vi "TreeItem.Property.Set.vi"(4 "Set String as Binary":bool, 6 "Custom Device Path":string, 8 "error in (no error)":errorcluster, 9 "Value":variant, 10 "Property Name":string, 11 "BaseNodeType":refnum<k24>) -> (0 "error out":errorcluster, 1 "Replaced":bool, 3 "BaseNodeType":refnum<k24>)   [LabVIEW 2016, in "Advanced System Definition.lvlib"]
doc: "Saves the new values/items into their corresponding position within the Custom Device Hierarchy according to their corresponding data type."
uses:
  SysDef API/Advanced System Definition.lvlib
  NationalInstruments.VeriStand.SystemStorage
  _Types/Property.DependentFile.ctl
  NationalInstruments.VeriStand
  <vilib>/NI Veristand/Custom Device API/Custom Device Item Ref.ctl
  NationalInstruments.VeriStand.SystemDefinitionAPI
  <vilib>/Utility/VariantDataType/VariantType.lvlib
  <vilib>/NI VeriStand/Custom Device API/Custom Device API.lvlib
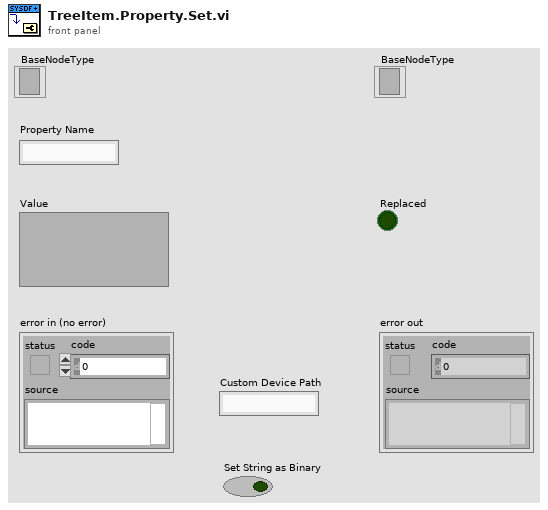
[diagram p1: front panel]
types:
  T1 = typedef "Advanced System Definition.lvlib/Property.DependentFile.ctl" = cluster{"Original Path":path, "Version":string, "RTDestination":path, "ForceDownload":bool, "SupportedTarget":string, "MD5":string}
  T2 = typedef "Custom Device API.lvlib/Custom Device Item Ref.ctl" = u64
  T3 = typedef "VariantType.lvlib/Type.ctl" = enum8{"Invalid Type", "Void", "I8", "I16", "I32", "I64", "U8", "U16", "U32", "U64", "Single Float", "Double Float", "Extended Float", "Single Complex", "Double Complex", "Extended Complex", "Enum U8", "Enum U16", "Enum U32", "Enum U64", "Single Float With Unit", "Double Float With Unit", "Extended Float With Unit", "Single Complex with Unit", "Double Complex with Unit", "Extended Complex with Unit", "Boolean", "String", "Path", "Picture", "Tag", "Array", "Cluster", "Variant", "LV Variant", "Waveform", "Timestamp", "Digital Waveform", "Digital Data", "ExpressData", "Refnum", "External Data", "VI", "Poly VI", "LabVIEW Class Instance", "Fixed Point"}
  T4 = typedef "Advanced System Definition.lvlib/Property.Dictionary.ctl" = cluster{"Dictionary Type":string, "Keys":string[], "Values":variant[]}
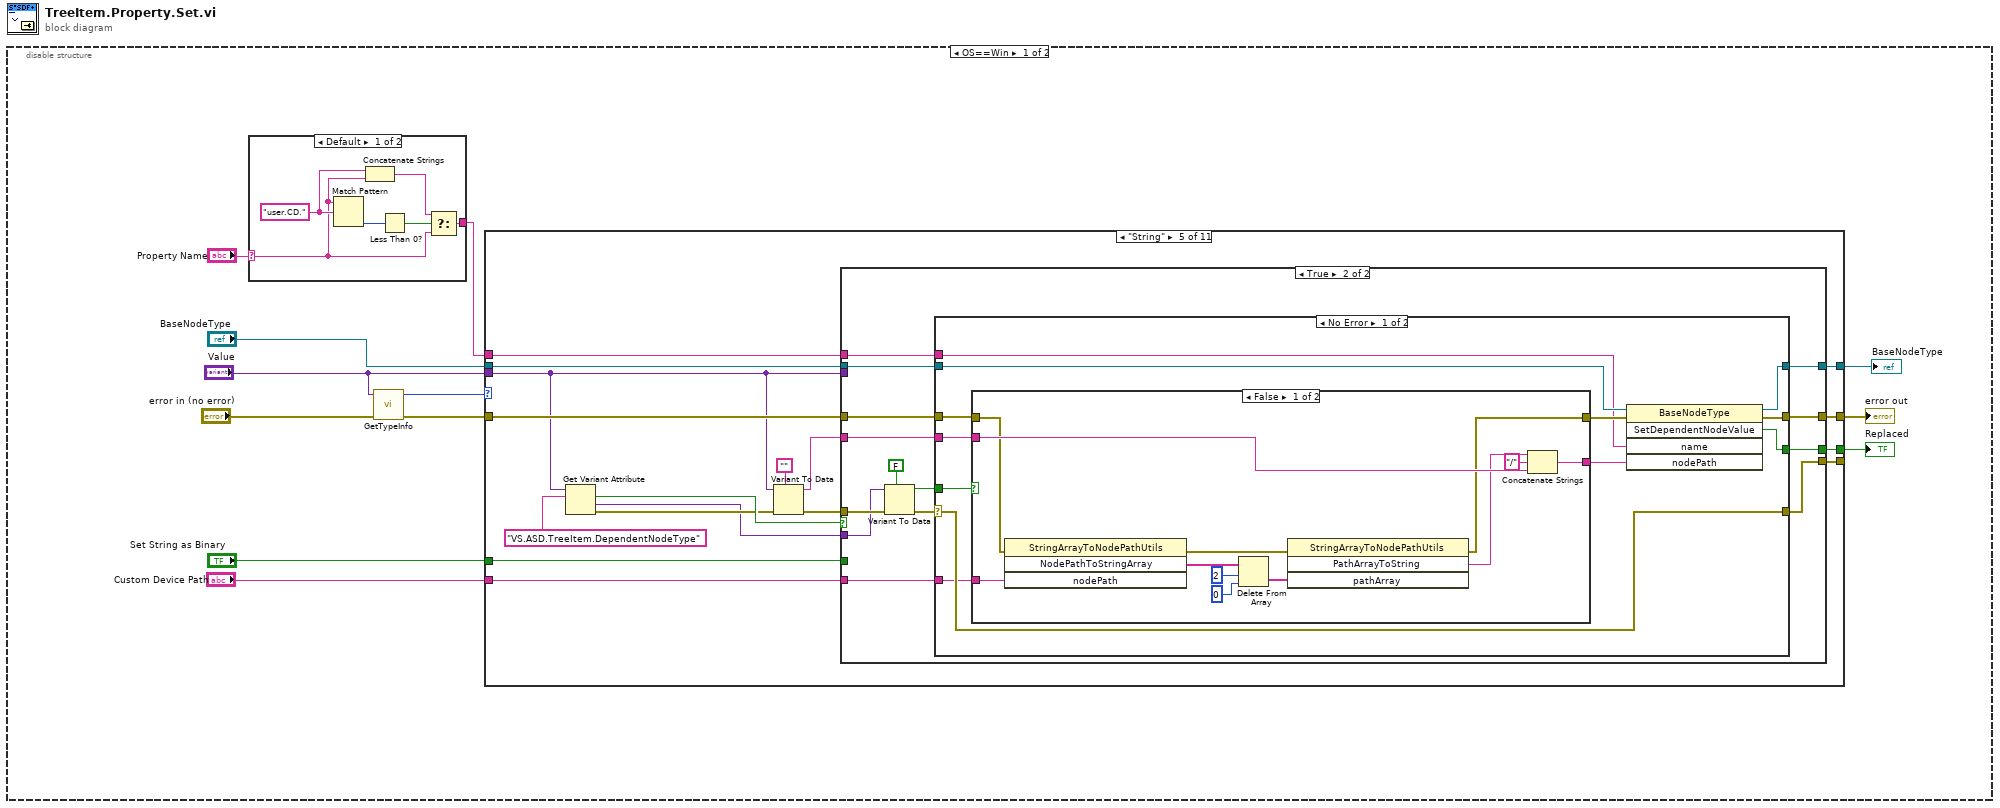
[diagram p0: block diagram]
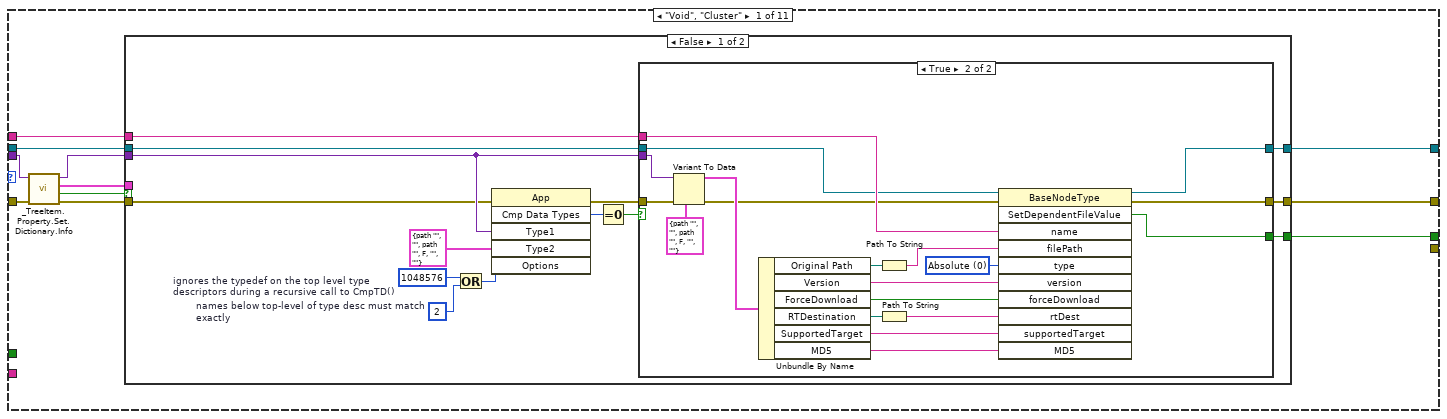
[diagram p3: hidden frame]
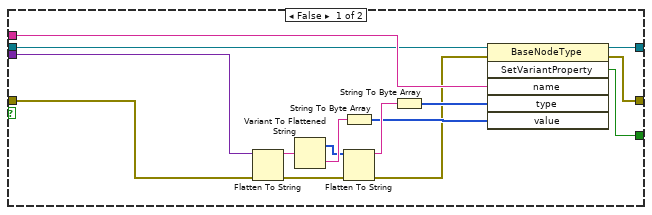
[diagram p4: hidden frame]
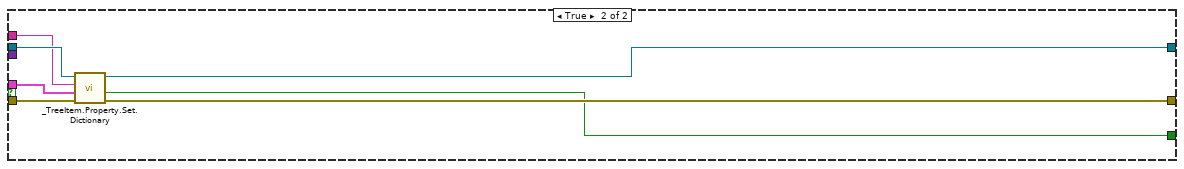
[diagram p5: hidden frame]
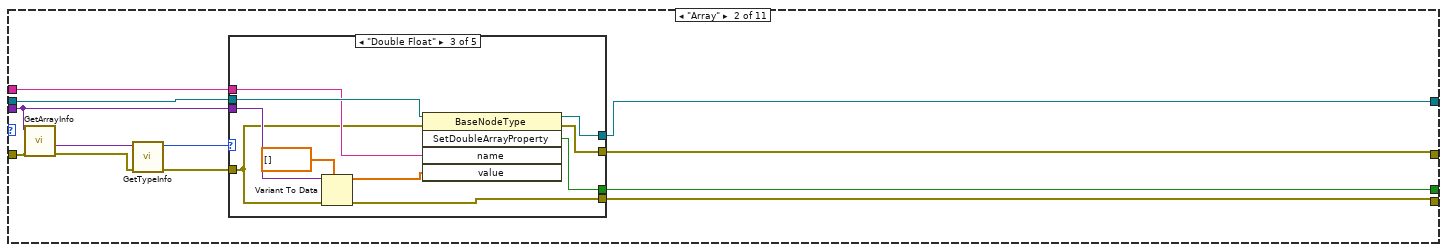
[diagram p6: hidden frame]
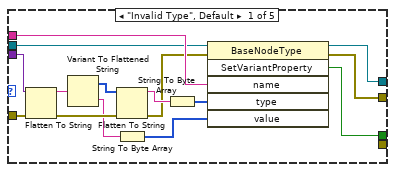
[diagram p7: hidden frame]
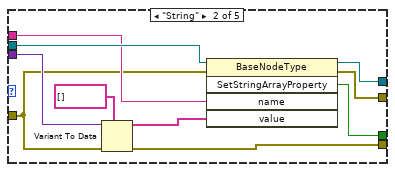
[diagram p8: hidden frame]
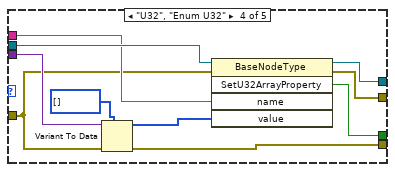
[diagram p9: hidden frame]
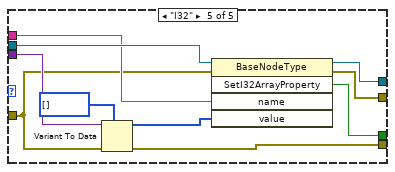
[diagram p10: hidden frame]
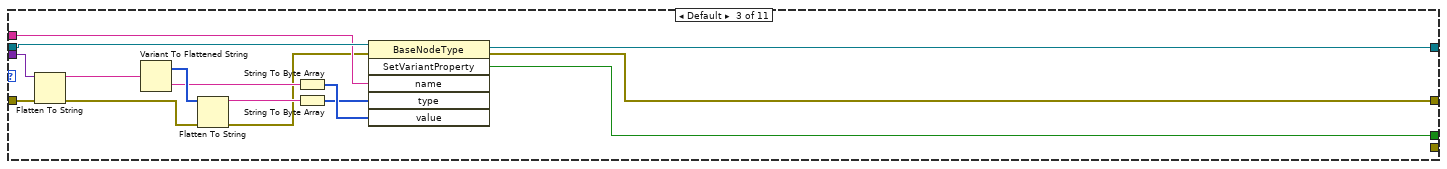
[diagram p11: hidden frame]
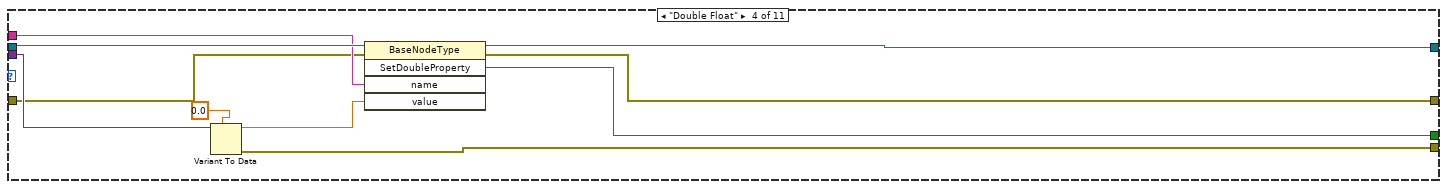
[diagram p12: hidden frame]
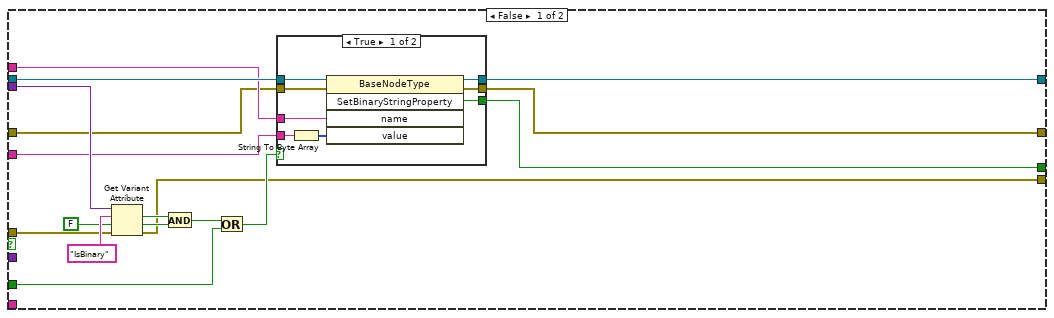
[diagram p13: hidden frame]
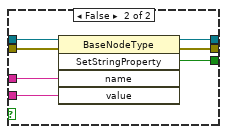
[diagram p14: hidden frame]
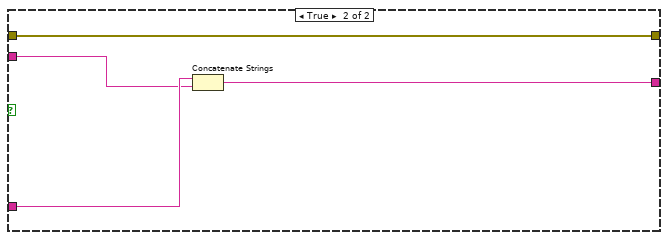
[diagram p15: hidden frame]
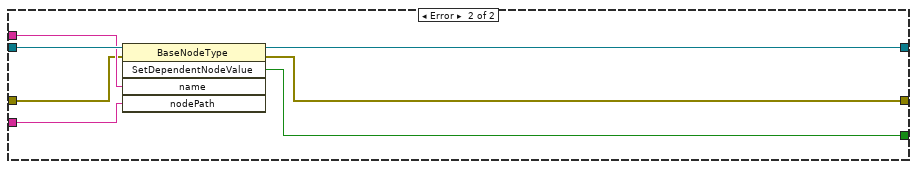
[diagram p16: hidden frame]
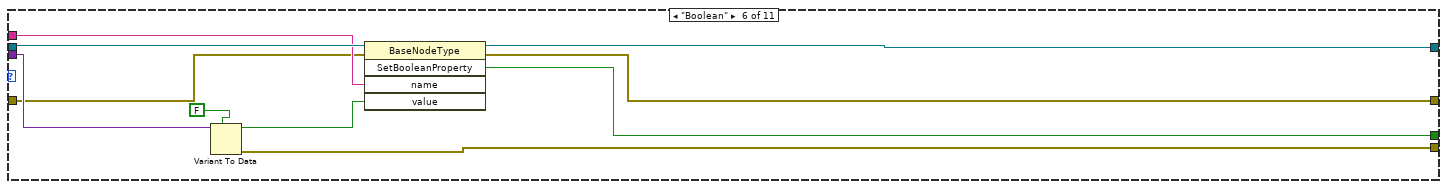
[diagram p17: hidden frame]
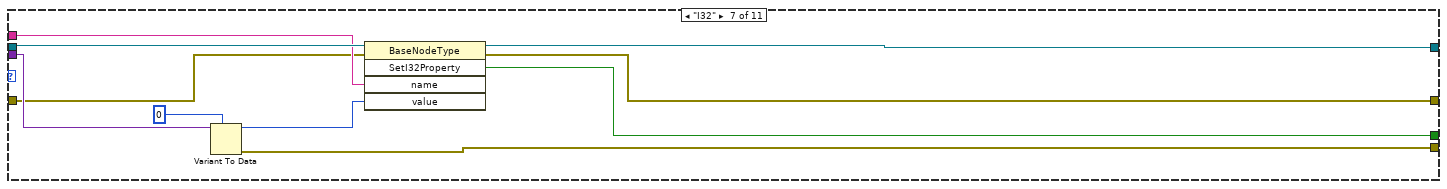
[diagram p18: hidden frame]
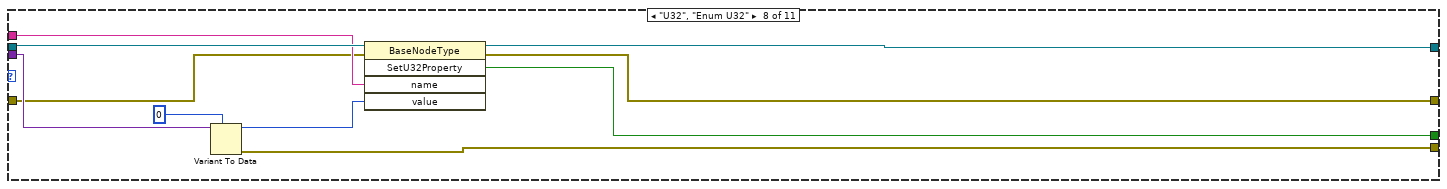
[diagram p19: hidden frame]
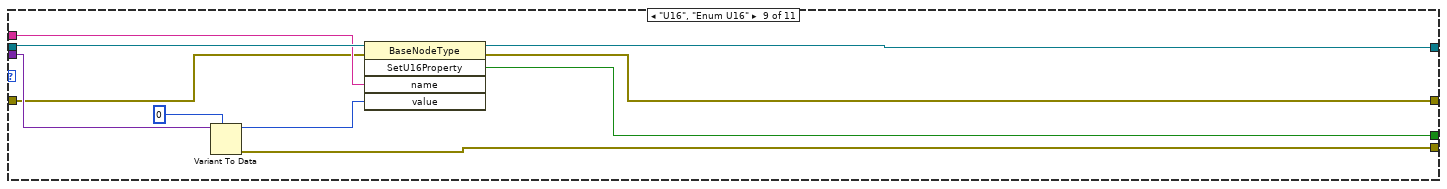
[diagram p20: hidden frame]
diagram:
  n1 = disable-structure shown="OS==Win" {
    frame condition #0 (active) {
      n2 = case shown="Default" "Property Name" {
        selector: "Property Name" -> [w13 w19]
        tunnel: [w14 w19] -> w3
        frame Default {
          w15 = "user.CD." ("regular expression")
          n3 = Match Pattern(string=w13, regular expression=w15) -> (offset past match=w18:i32)  [unwired: 1 in, 3 out]
          n4 = Concatenate Strings(w15, w13) -> (w16:string)
          n5 = Less Than 0?(x=w18) -> (x < 0?=w17:bool)
          n6 = Select(t=w16, s=w17, f=w13) -> (s? t:f=w14:string)
        }
        frame "Value Table" {
        }
      }
      n7 = call <vilib>:"GetTypeInfo.vi"("error in (no error)"="error in (no error)", "Variant"="Value") -> ("error out"=w8:errorcluster, "Type Enum"=w12:T3)  [unwired: 5 in, 3 out]
      n8 = case shown="\"String\"" w12 {
        tunnel: "BaseNodeType" -> [w29 w92 w167 w174 w193 w282 w292 w302 w312 w319 w356]
        tunnel: w8 -> [w24 w97 w157 w172 w186 w280 w290 w300 w310 w322 w355]
        tunnel: [w28 w90 w165 w171 w191 w279 w289 w299 w309 w318 w351] -> w11
        tunnel: w3 -> [w30 w91 w166 w173 w192 w281 w291 w301 w311 w320 w353]
        tunnel: "Value" -> [w25 w86 w156 w177 w181 w285 w295 w305 w315 w328 w359]
        tunnel: [w27 w89 w164 w170 w190 w278 w288 w298 w308 w316 w350] -> w10
        tunnel: [_ w88 _ w175 w194 w283 w293 w303 w313 _ w354] -> _
        tunnel: [w26 w87 w163 w168 w189 w276 w286 w296 w306 w317 w349] -> w5
        tunnel: "Set String as Binary" -> [_ _ _ _ w188 _ _ _ _ _ _]
        tunnel: "Custom Device Path" -> [_ _ _ _ w178 _ _ _ _ _ _]
        frame "Void", "Cluster" {
          n9 = call "_TreeItem.Property.Set.Dictionary.Info.vi"("error in"=w24, "Variant"=w25) -> ("error out"=w23:errorcluster, "Dictionary?"=w22:bool, "Dictionary Info"=w21:T4, "Variant out"=w20:variant)  [unwired: 6 in]
          n10 = case shown="False" w22 {
            tunnel: w30 -> [w44 w84]
            tunnel: w29 -> [w43 w85]
            tunnel: [w42 w82] -> w28
            tunnel: [w41 w80] -> w27
            tunnel: [w40 w81] -> w26
            tunnel: w20 -> [w35 _]
            tunnel: w23 -> [w32 w83]
            tunnel: w21 -> [_ w79]
            frame False {
              w38 = 2  # names below top-level of type desc must match exactly
              w37 = 1048576  # ignores the typedef on the top level type descriptors during a recursive call to CmpTD()
              n11 = Or(x=w37, y=w38) -> (x .or. y?=w39:i32)
              n12 = invoke class="App" method="Cmp Data Types"(error in=w32, "Type1"=w35, "Type2"=T1 {"Original Path"=path "", "Version"="", "RTDestination"=path "", "ForceDownload"=FALSE, "SupportedTarget"="", "MD5"=""} ("OptionalInfo"), "Options"=w39) -> (error out=w31:errorcluster, "Compare Data Types"=w36:i32)  [unwired: 2 in, 4 out]
              n13 = Equal To 0?(x=w36) -> (x = 0?=w33:bool)
              n14 = case shown="True" w33 {
                tunnel: w44 -> [w59 w73]
                tunnel: w43 -> [w58 w71]
                tunnel: [w57 w62] -> w42
                tunnel: [w56 w61] -> w41
                tunnel: [w55 w70] -> w40
                tunnel: w31 -> [w49 w77]
                tunnel: w35 -> [w45 w78]
                frame False {
                  n15 = Flatten To String(anything=w45, error in (no error)=w49) -> (data string=w51:string, error out=w50:errorcluster)  [unwired: 2 in, 1 out]
                  n16 = Variant To Flattened String(Variant=w51) -> (data string=w54:string, 1:w52:i16[])
                  n17 = String To Byte Array(string=w54) -> (unsigned byte array=w48:u8[])
                  n18 = Flatten To String(anything=w52, error in (no error)=w50) -> (data string=w53:string, error out=w46:errorcluster)  [unwired: 2 in, 1 out]
                  n19 = String To Byte Array(string=w53) -> (unsigned byte array=w47:u8[])
                  n20 = invoke class="BaseNodeType" method="SetVariantProperty"(reference=w58, error in=w46, "name"=w59, "type"=w47, "value"=w48) -> (reference out=w55:refnum<k24>, error out=w57:errorcluster, "SetVariantProperty"=w56:bool)  [unwired: 1 in, 3 out]
                }
                frame True {
                  w60 = 0 items=["Absolute", "Relative", "ToCommonDocDir", "ToApplicationDataDir"] ("type")
                  n21 = Variant To Data(error in=w77, type=T1 {"Original Path"=path "", "Version"="", "RTDestination"=path "", "ForceDownload"=FALSE, "SupportedTarget"="", "MD5"=""} ("OptionalInfo"), Variant=w78) -> (data=w74:T1, error out=w63:errorcluster)
                  n22 = Unbundle By Name(w74) -> ("Original Path"=w72:path, "Version"=w68:string, "ForceDownload"=w67:bool, "RTDestination"=w75:path, "SupportedTarget"=w65:string, "MD5"=w64:string)
                  n23 = Path To String(path=w72) -> (string=w69:string)
                  n24 = Path To String(path=w75) -> (string=w66:string)
                  n25 = invoke class="BaseNodeType" method="SetDependentFileValue"(reference=w71, error in=w63, "name"=w73, "filePath"=w69, "type"=w60, "version"=w68, "forceDownload"=w67, "rtDest"=w66, "supportedTarget"=w65, "MD5"=w64) -> (reference out=w70:refnum<k24>, error out=w62:errorcluster, "SetDependentFileValue"=w61:bool)  [unwired: 1 in, 8 out]
                }
              }
            }
            frame True {
              n26 = call "_TreeItem.Property.Set.Dictionary.vi"("error in (no error)"=w83, "Dictionary"=w79, "Property Name"=w84, "BaseNodeType"=w85) -> ("error out"=w82:errorcluster, "Replaced"=w80:bool, "BaseNodeType out"=w81:refnum<k24>)  [unwired: 5 in]
            }
          }
        }
        frame "Array" {
          n27 = call <vilib>:"GetArrayInfo.vi"("error in (no error)"=w97, "Variant"=w86) -> ("error out"=w95:errorcluster, "ArrayElement"=w96:variant)  [unwired: 6 in, 2 out]
          n28 = call <vilib>:"GetTypeInfo.vi"("error in (no error)"=w95, "Variant"=w96) -> ("error out"=w93:errorcluster, "Type Enum"=w94:T3)  [unwired: 5 in, 3 out]
          n29 = case shown="\"Double Float\"" w94 {
            tunnel: w93 -> [w99 w115 w127 w136 w147]
            tunnel: w86 -> [w100 w122 w132 w142 w152]
            tunnel: w92 -> [w111 w119 w130 w140 w150]
            tunnel: w91 -> [w112 w117 w128 w138 w148]
            tunnel: [w110 w118 w129 w139 w149] -> w87
            tunnel: [w109 w113 w125 w134 w145] -> w90
            tunnel: [w108 w114 w126 w135 w146] -> w89
            tunnel: [_ w120 w131 w141 w151] -> w88
            frame "Invalid Type", Default {
              n30 = Flatten To String(anything=w100, error in (no error)=w99) -> (data string=w106:string, error out=w107:errorcluster)  [unwired: 2 in, 1 out]
              n31 = Variant To Flattened String(Variant=w106) -> (data string=w103:string, 1:w105:i16[])
              n32 = Flatten To String(anything=w105, error in (no error)=w107) -> (data string=w104:string, error out=w98:errorcluster)  [unwired: 2 in, 1 out]
              n33 = String To Byte Array(string=w103) -> (unsigned byte array=w101:u8[])
              n34 = String To Byte Array(string=w104) -> (unsigned byte array=w102:u8[])
              n35 = invoke class="BaseNodeType" method="SetVariantProperty"(reference=w111, error in=w98, "name"=w112, "type"=w102, "value"=w101) -> (reference out=w110:refnum<k24>, error out=w109:errorcluster, "SetVariantProperty"=w108:bool)  [unwired: 1 in, 3 out]
            }
            frame "String" {
              n36 = Variant To Data(error in=w115, type=string[] [], Variant=w122) -> (data=w116:string[], error out=w120:errorcluster)
              n37 = invoke class="BaseNodeType" method="SetStringArrayProperty"(reference=w119, error in=w115, "name"=w117, "value"=w116) -> (reference out=w118:refnum<k24>, error out=w113:errorcluster, "SetStringArrayProperty"=w114:bool)  [unwired: 1 in, 2 out]
            }
            frame "Double Float" {
              n38 = Variant To Data(error in=w127, type=dbl[] [], Variant=w132) -> (data=w123:dbl[], error out=w131:errorcluster)
              n39 = invoke class="BaseNodeType" method="SetDoubleArrayProperty"(reference=w130, error in=w127, "name"=w128, "value"=w123) -> (reference out=w129:refnum<k24>, error out=w125:errorcluster, "SetDoubleArrayProperty"=w126:bool)  [unwired: 1 in, 2 out]
            }
            frame "U32", "Enum U32" {
              n40 = Variant To Data(error in=w136, type=u32[] [], Variant=w142) -> (data=w137:u32[], error out=w141:errorcluster)
              n41 = invoke class="BaseNodeType" method="SetU32ArrayProperty"(reference=w140, error in=w136, "name"=w138, "value"=w137) -> (reference out=w139:refnum<k24>, error out=w134:errorcluster, "SetU32ArrayProperty"=w135:bool)  [unwired: 1 in, 2 out]
            }
            frame "I32" {
              n42 = Variant To Data(error in=w147, type=i32[] [], Variant=w152) -> (data=w143:i32[], error out=w151:errorcluster)
              n43 = invoke class="BaseNodeType" method="SetI32ArrayProperty"(reference=w150, error in=w147, "name"=w148, "value"=w143) -> (reference out=w149:refnum<k24>, error out=w145:errorcluster, "SetI32ArrayProperty"=w146:bool)  [unwired: 1 in, 2 out]
            }
          }
        }
        frame Default {
          n44 = Flatten To String(anything=w156, error in (no error)=w157) -> (data string=w161:string, error out=w162:errorcluster)  [unwired: 2 in, 1 out]
          n45 = Variant To Flattened String(Variant=w161) -> (data string=w158:string, 1:w160:i16[])
          n46 = Flatten To String(anything=w160, error in (no error)=w162) -> (data string=w159:string, error out=w155:errorcluster)  [unwired: 2 in, 1 out]
          n47 = String To Byte Array(string=w158) -> (unsigned byte array=w154:u8[])
          n48 = String To Byte Array(string=w159) -> (unsigned byte array=w153:u8[])
          n49 = invoke class="BaseNodeType" method="SetVariantProperty"(reference=w167, error in=w155, "name"=w166, "type"=w153, "value"=w154) -> (reference out=w163:refnum<k24>, error out=w165:errorcluster, "SetVariantProperty"=w164:bool)  [unwired: 1 in, 3 out]
        }
        frame "Double Float" {
          n50 = Variant To Data(type=0.0, Variant=w177) -> (data=w169:dbl, error out=w175:errorcluster)  [unwired: 1 in]
          n51 = invoke class="BaseNodeType" method="SetDoubleProperty"(reference=w174, error in=w172, "name"=w173, "value"=w169) -> (reference out=w168:refnum<k24>, error out=w171:errorcluster, "SetDoubleProperty"=w170:bool)  [unwired: 1 in, 2 out]
        }
        frame "String" {
          n52 = Get Variant Attribute(Variant=w181, name="VS.ASD.TreeItem.DependentNodeType") -> (found=w185:bool, value=w179:variant, error out=w183:errorcluster)  [unwired: 2 in, 1 out]
          n53 = Variant To Data(error in=w183, type="", Variant=w181) -> (data=w180:string, error out=w182:errorcluster)
          n54 = case shown="True" w185 {
            tunnel: [w195 w229] -> w194
            tunnel: w193 -> [w211 w240]
            tunnel: w192 -> [w210 w238]
            tunnel: [w209 w236] -> w191
            tunnel: [w208 w235] -> w190
            tunnel: [w207 w239] -> w189
            tunnel: w188 -> [w201 _]
            tunnel: w181 -> [w199 _]
            tunnel: w182 -> [w198 w233]
            tunnel: w186 -> [w197 w237]
            tunnel: w180 -> [w196 w234]
            tunnel: w179 -> [_ w232]
            tunnel: w178 -> [_ w227]
            frame False {
              n55 = Get Variant Attribute(Variant=w199, name="IsBinary", default value (empty Variant)=FALSE ("Set String as Binary"), error in=w198) -> (found=w204:bool, value=w205:bool, error out=w195:errorcluster)  [unwired: 1 out]
              n56 = And(x=w204, y=w205) -> (x .and. y?=w206:bool)
              n57 = Or(x=w206, y=w201) -> (x .or. y?=w200:bool)
              n58 = case shown="True" w200 {
                tunnel: w211 -> [w219 w226]
                tunnel: w210 -> [w218 w225]
                tunnel: w197 -> [w217 w224]
                tunnel: [w216 w223] -> w209
                tunnel: [w215 w222] -> w208
                tunnel: w196 -> [w214 w221]
                tunnel: [w213 w220] -> w207
                frame True {
                  n59 = String To Byte Array(string=w214) -> (unsigned byte array=w212:u8[])
                  n60 = invoke class="BaseNodeType" method="SetBinaryStringProperty"(reference=w219, error in=w217, "name"=w218, "value"=w212) -> (reference out=w213:refnum<k24>, error out=w216:errorcluster, "SetBinaryStringProperty"=w215:bool)  [unwired: 1 in, 2 out]
                }
                frame False {
                  n61 = invoke class="BaseNodeType" method="SetStringProperty"(reference=w226, error in=w224, "name"=w225, "value"=w221) -> (reference out=w220:refnum<k24>, error out=w223:errorcluster, "SetStringProperty"=w222:bool)  [unwired: 1 in, 2 out]
                }
              }
            }
            frame True {
              n62 = Variant To Data(error in=w233, type=FALSE, Variant=w232) -> (data=w228:bool, error out=w231:errorcluster)
              n63 = case shown="No Error" w231 {
                selector: w231 -> [w252 _]
                tunnel: w240 -> [w245 w275]
                tunnel: [w246 w274] -> w239
                tunnel: w238 -> [w244 w273]
                tunnel: w237 -> [w251 w272]
                tunnel: [w247 w271] -> w236
                tunnel: [w242 w270] -> w235
                tunnel: w234 -> [w250 w269]
                tunnel: [w252 _] -> w229
                tunnel: w228 -> [w249 _]
                tunnel: w227 -> [w241 _]
                frame No Error {
                  n64 = case shown="False" w249 {
                    tunnel: w241 -> [w260 w268]
                    tunnel: w250 -> [w259 w267]
                    tunnel: [w257 w266] -> w243
                    tunnel: w251 -> [w253 w265]
                    tunnel: [w254 w265] -> w248
                    frame False {
                      n65 = invoke class="StringArrayToNodePathUtils" method="NodePathToStringArray"(error in=w253, "nodePath"=w260) -> (error out=w261:errorcluster, "NodePathToStringArray"=w264:string[])  [unwired: 2 in, 2 out]
                      n66 = Delete From Array(array=w264, length=2, index=0) -> (deleted portion=w255:string[])  [unwired: 1 out]
                      n67 = invoke class="StringArrayToNodePathUtils" method="PathArrayToString"(error in=w261, "pathArray"=w255) -> (error out=w254:errorcluster, "PathArrayToString"=w258:string)  [unwired: 2 in, 2 out]
                      n68 = Concatenate Strings(w258, "/" ("string"), w259) -> (w257:string)
                    }
                    frame True {
                      n69 = Concatenate Strings(w268, w267) -> (w266:string)
                    }
                  }
                  n70 = invoke class="BaseNodeType" method="SetDependentNodeValue"(reference=w245, error in=w248, "name"=w244, "nodePath"=w243) -> (reference out=w246:refnum<k24>, error out=w247:errorcluster, "SetDependentNodeValue"=w242:bool)  [unwired: 1 in, 2 out]
                }
                frame Error {
                  n71 = invoke class="BaseNodeType" method="SetDependentNodeValue"(reference=w275, error in=w272, "name"=w273, "nodePath"=w269) -> (reference out=w274:refnum<k24>, error out=w271:errorcluster, "SetDependentNodeValue"=w270:bool)  [unwired: 1 in, 2 out]
                }
              }
            }
          }
        }
        frame "Boolean" {
          n72 = Variant To Data(type=FALSE, Variant=w285) -> (data=w277:bool, error out=w283:errorcluster)  [unwired: 1 in]
          n73 = invoke class="BaseNodeType" method="SetBooleanProperty"(reference=w282, error in=w280, "name"=w281, "value"=w277) -> (reference out=w276:refnum<k24>, error out=w279:errorcluster, "SetBooleanProperty"=w278:bool)  [unwired: 1 in, 2 out]
        }
        frame "I32" {
          n74 = Variant To Data(type=0, Variant=w295) -> (data=w287:i32, error out=w293:errorcluster)  [unwired: 1 in]
          n75 = invoke class="BaseNodeType" method="SetI32Property"(reference=w292, error in=w290, "name"=w291, "value"=w287) -> (reference out=w286:refnum<k24>, error out=w289:errorcluster, "SetI32Property"=w288:bool)  [unwired: 1 in, 2 out]
        }
        frame "U32", "Enum U32" {
          n76 = Variant To Data(type=u32 0, Variant=w305) -> (data=w297:u32, error out=w303:errorcluster)  [unwired: 1 in]
          n77 = invoke class="BaseNodeType" method="SetU32Property"(reference=w302, error in=w300, "name"=w301, "value"=w297) -> (reference out=w296:refnum<k24>, error out=w299:errorcluster, "SetU32Property"=w298:bool)  [unwired: 1 in, 2 out]
        }
        frame "U16", "Enum U16" {
          n78 = Variant To Data(type=u16 0, Variant=w315) -> (data=w307:u16, error out=w313:errorcluster)  [unwired: 1 in]
          n79 = invoke class="BaseNodeType" method="SetU16Property"(reference=w312, error in=w310, "name"=w311, "value"=w307) -> (reference out=w306:refnum<k24>, error out=w309:errorcluster, "SetU16Property"=w308:bool)  [unwired: 1 in, 2 out]
        }
        frame "U64" {
          # "This is the legacy dependent node format;\ndependent node properties are now serialized\nas strings containing the node path with a variant\nattribute to indicate they are dependent nodes."
          n80 = Variant To Data(error in=w322, type=u64 0, Variant=w328) -> (data=w323:u64)  [unwired: 1 out]
          n81 = Equal?(x=T2 18446744073709551615 ("Dependent Node Ref"), y=w323) -> (x = y?=w325:bool)
          n82 = case shown="False" w325 {
            tunnel: [w338 ""] -> w324
            tunnel: w323 -> [w331 _]
            tunnel: w322 -> [w330 w347]
            tunnel: [w329 w347] -> w321
            frame False {
              n83 = constructor class="NodeIDUtil"(error in=w330) -> (reference out=w334:refnum<k24>, error out=w335:errorcluster)  [unwired: 2 in, 1 out]
              n84 = invoke class="NodeIDUtil" method="IDToBaseNode"(reference=w334, error in=w335, "nodeID"=w331) -> (reference out=w337:refnum<k24>, error out=w336:errorcluster, "IDToBaseNode"=w332:refnum<k24>)  [unwired: 1 in, 1 out]
              n85 = Close Reference(reference=w337, error in (no error)=w336) -> (error out=w333:errorcluster)
              n86 = case shown="No Error" w333 {
                selector: w333 -> [w340 w345]
                tunnel: w332 -> [w344 _]
                tunnel: [w343 ""] -> w338
                tunnel: [w339 w345] -> w329
                frame No Error {
                  n87 = property class="BaseNode"(reference=w344, error in=w340) -> (reference out=w341:refnum<k24>, error out=w342:errorcluster, "NodePath"=w343:string)
                  n88 = Close Reference(reference=w341, error in (no error)=w342) -> (error out=w339:errorcluster)
                }
                frame Error {
                }
              }
            }
            frame True {
              # "If user call this with an invalid pointer, we will\nset this to an empty node path."
            }
          }
          n89 = invoke class="BaseNodeType" method="SetDependentNodeValue"(reference=w319, error in=w321, "name"=w320, "nodePath"=w324) -> (reference out=w317:refnum<k24>, error out=w318:errorcluster, "SetDependentNodeValue"=w316:bool)  [unwired: 1 in, 2 out]
        }
        frame "Path" {
          n90 = Variant To Data(type=path "", Variant=w359) -> (data=w357:path, error out=w354:errorcluster)  [unwired: 1 in]
          n91 = Path To String(path=w357) -> (string=w352:string)
          n92 = invoke class="BaseNodeType" method="SetStringProperty"(reference=w356, error in=w355, "name"=w353, "value"=w352) -> (reference out=w349:refnum<k24>, error out=w351:errorcluster, "SetStringProperty"=w350:bool)  [unwired: 1 in, 2 out]
        }
      }
      "Replaced" <- w10
      "error out" <- w11
      "BaseNodeType" <- w5
    }
    frame condition #1 {
    }
  }
